vi "Deploy to Platform.vi"(8 "error in (no error)":errorcluster, 9 "VIA":string, 10 "Platform":string, 11 "TargetPluginManager in":refnum<class "TargetPluginManager.lvclass">) -> (0 "error out":errorcluster, 1 "Processed VIA":string, 2 "Deployed Resource":string, 3 "TargetPluginManager out":refnum<class "TargetPluginManager.lvclass">, 5 "Response":string)   [LabVIEW 2020, in "PicoG-Core.lvlib" / "TargetPluginManager.lvclass"]
uses:
  TargetPluginManager.lvclass
  DeployResource/DeployResource.lvclass
  DeployTarget/DeployTarget.lvclass
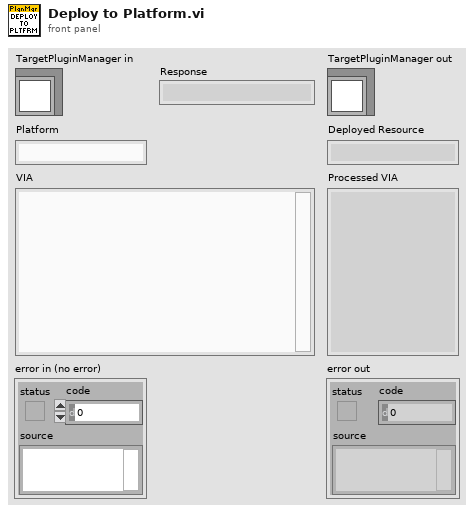
[diagram p1: front panel]
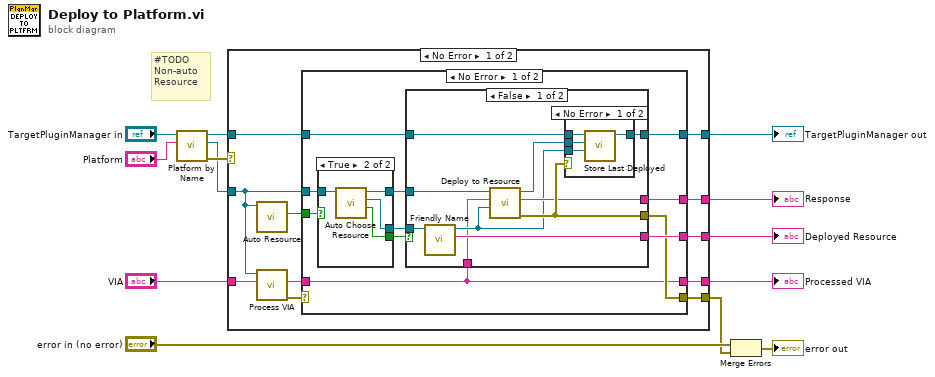
[diagram p0: block diagram]
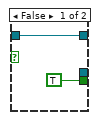
[diagram p2: hidden frame]
diagram:
  # "#TODO\nNon-auto Resource"
  n1 = call "Platform by Name.vi"("Platform"="Platform", "TargetPluginManager in"="TargetPluginManager in") -> ("error out"=w9:errorcluster, "Target"=w1:refnum<class "DeployTarget.lvclass">, "TargetPluginManager out"=w10:refnum<class "TargetPluginManager.lvclass">)  [unwired: 7 in]
  n2 = case shown="No Error" w9 {
    selector: w9 -> [_ w61]
    tunnel: w10 -> [w17 w60]
    tunnel: w1 -> [w22 _]
    tunnel: "VIA" -> [w24 _]
    tunnel: [w19 w61] -> w6
    tunnel: [w21 w60] -> w5
    tunnel: [w14 _] -> w4
    tunnel: [w20 _] -> w3
    tunnel: [w18 _] -> w2
    frame No Error {
      n3 = call-dynamic "Auto Resource.vi"("DeployTarget in"=w22) -> ("Auto Resource"=w23:bool)  [unwired: 8 in, 2 out]
      n4 = call-dynamic "Process VIA.vi"("Raw VIA"=w24, "DeployTarget in"=w22) -> ("error out"=w16:errorcluster, "VIA"=w15:string)  [unwired: 7 in, 1 out]
      n5 = case shown="No Error" w16 {
        selector: w16 -> [_ w59]
        tunnel: w23 -> [w35 _]
        tunnel: w22 -> [w34 _]
        tunnel: [w31 w58] -> w21
        tunnel: [w30 _] -> w20
        tunnel: w15 -> [w25 _]
        tunnel: [w28 w59] -> w19
        tunnel: [w27 _] -> w18
        tunnel: w17 -> [w26 w58]
        tunnel: [w25 _] -> w14
        frame No Error {
          n6 = case shown="True" w35 {
            tunnel: w34 -> [w36 w39]
            tunnel: [_ w41] -> w33
            tunnel: [TRUE ("Cancelled") w40] -> w32
            tunnel: [w36 w38] -> w29
            frame False {
            }
            frame True {
              n7 = call-dynamic "Auto Choose Resource.vi"("DeployTarget in"=w39) -> ("Cancelled"=w40:bool, "Resource"=w41:refnum<class "DeployResource.lvclass">, "DeployTarget out"=w38:refnum<class "DeployTarget.lvclass">)  [unwired: 7 in, 1 out]
            }
          }
          n8 = case shown="False" w32 {
            tunnel: w33 -> [w50 _]
            tunnel: w26 -> [w47 w57]
            tunnel: [w46 w57] -> w31
            tunnel: [w49 _] -> w30
            tunnel: w29 -> [w45 _]
            tunnel: w25 -> [w42 _]
            tunnel: [w51 _] -> w28
            tunnel: [w48 _] -> w27
            frame False {
              n9 = call-dynamic "Friendly Name.vi"("DeployResource in"=w50) -> ("Friendly Name"=w49:string, "DeployResource out"=w43:refnum<class "DeployResource.lvclass">)  [unwired: 8 in, 1 out]
              n10 = call-dynamic "Deploy to Resource.vi"("Resource"=w43, "VIA"=w42, "DeployTarget in"=w45) -> ("error out"=w51:errorcluster, "Response"=w48:string, "DeployTarget out"=w44:refnum<class "DeployTarget.lvclass">)  [unwired: 6 in]
              n11 = case shown="No Error" w51 {
                tunnel: w47 -> [w55 w56]
                tunnel: [w54 w56] -> w46
                tunnel: w43 -> [w53 _]
                tunnel: w44 -> [w52 _]
                frame No Error {
                  n12 = call "Store Last Deployed.vi"("PicoG-Core:DeployResource"=w53, "PicoG-Core:DeployTarget"=w52, "TargetPluginManager in"=w55) -> ("TargetPluginManager out"=w54:refnum<class "TargetPluginManager.lvclass">)  [unwired: 7 in, 1 out]
                }
                frame Error {
                }
              }
            }
            frame True {
            }
          }
        }
        frame Error {
        }
      }
    }
    frame Error {
    }
  }
  "TargetPluginManager out" <- w5
  "Processed VIA" <- w4
  "Deployed Resource" <- w3
  "Response" <- w2
  n13 = Merge Errors("error in (no error)", w6) -> (→"error out":errorcluster)
